vi "INIT SetDBAliasProperty.vi"(7 "DB Alias data":T1, 8 "error in (no error)":errorcluster, 11 "Device Item Ref in":T2 format="%.0x") -> (0 "error out":errorcluster, 3 "Device Item Ref out":T2 format="%.0x")   [LabVIEW 2018, in "CAN Gateway System Explorer.lvlib"]
uses:
  CAN Gateway System Explorer.lvlib
  <vilib>/NI Veristand/Custom Device API/Custom Device Item Ref.ctl
  Types/Alias DB data.ctl
  Shared/Constants.vi
  <vilib>/NI Veristand/Custom Device API/Set Item Property (String).vi
  <vilib>/NI Veristand/Custom Device API/Custom Device API.lvlib
  Shared/CAN Gateway Shared.lvlib
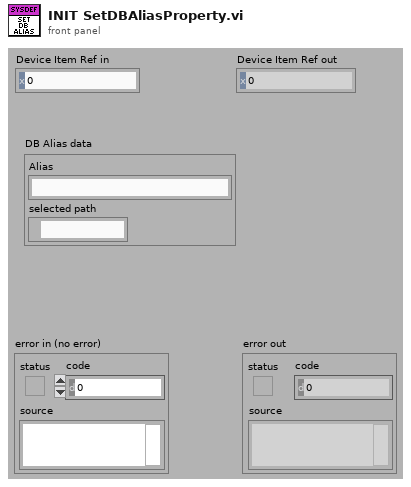
[diagram p1: front panel]
types:
  T1 = typedef "CAN Gateway System Explorer.lvlib/Alias DB data.ctl" = cluster{"Alias":string, "selected path":path}
  T2 = typedef "Custom Device API.lvlib/Custom Device Item Ref.ctl" = u64
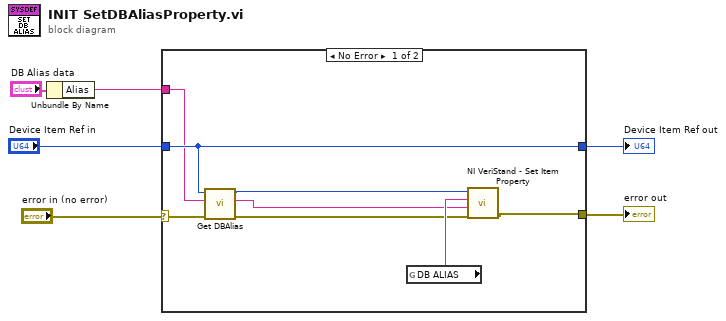
[diagram p0: block diagram]
diagram:
  n1 = Unbundle By Name("DB Alias data") -> ("Alias"=w1:string)
  n2 = case shown="No Error" "error in (no error)" {
    selector: "error in (no error)" -> [w14 w16]
    tunnel: [w12 w16] -> w6
    tunnel: [w11 w15] -> w4
    tunnel: "Device Item Ref in" -> [w11 w15]
    tunnel: w1 -> [w8 _]
    frame No Error {
      n3 = call "Get DBAlias.vi"("error in (no error)"=w14, "DB Alias"=w8, "Device Item Ref in"=w11) -> ("error out"=w9:errorcluster, "Alias"=w7:string, "Device Item Ref out"=w10:T2)  [unwired: 6 in]
      n4 = global read "Constants.vi" "DB ALIAS"() -> (w13:string)
      n5 = call-poly <vilib>:"NI VeriStand - Set Item Property.vi"("error in (no error)"=w9, "Value"=w7, "Property Name"=w13, "Item Ref in"=w10) -> ("error out"=w12:errorcluster)  [unwired: 5 in, 2 out]
    }
    frame Error {
    }
  }
  "error out" <- w6
  "Device Item Ref out" <- w4
